vi "网分测量.vi"() -> (2 "Freq&S":T1)   [LabVIEW 2015]
uses:
  network_Global/Global.vi
  network/network.lvclass
  E5071C/Agilent ENA Series/Agilent ENA Series.lvlib
panel:
  in  "VISA resource name":refnum<visa-resource-name>
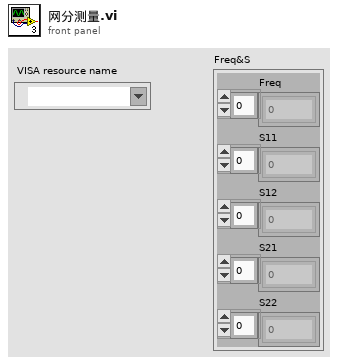
[diagram p1: front panel]
types:
  T1 = cluster{"Freq":dbl[], "S11":dbl[], "S12":dbl[], "S21":dbl[], "S22":dbl[]}
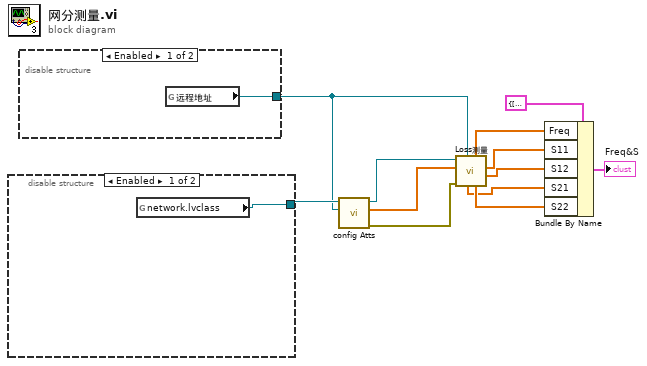
[diagram p0: block diagram]
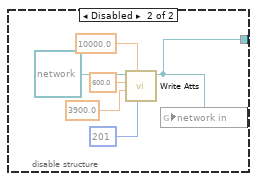
[diagram p2: hidden frame]
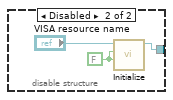
[diagram p3: hidden frame]
diagram:
  n1 = disable-structure shown="Enabled" {
    disable-tunnel: [w13 w14] -> w10
    frame Enabled {
      n2 = global read "Global.vi" "network.lvclass"() -> (w13:refnum<class "network.lvclass">)
    }
    frame Disabled {
      n3 = call-dynamic "Write Atts.vi"("Points"=201, "IF_Band"=10000.0, "Stop"=3900.0 ("Start"), "Start"=600.0, "network in"=refnum<class "network.lvclass"> refnum ("network.lvclass")) -> ("network out"=w14:refnum<class "network.lvclass">)  [unwired: 5 in, 1 out]
      n4 = global write "Global.vi" "network in"(w14) -> ()
    }
  }
  n5 = disable-structure shown="Enabled" {
    disable-tunnel: [w20 w21] -> w6
    frame Enabled {
      n6 = global read "Global.vi" "远程地址"() -> (w20:refnum<visa-resource-name>)
    }
    frame Disabled {
      w23 = FALSE ("Reset? (T: Yes)")
      n7 = call "Initialize.vi"("Reset? (T: Yes)"=w23, "ID Query? (T: Yes)"=w23, "VISA resource name"="VISA resource name") -> ("VISA resource name out"=w21:refnum<visa-resource-name>)  [unwired: 7 in, 1 out]
    }
  }
  n8 = call-dynamic "config Atts.vi"("VISA resource name"=w6, "network in"=w10) -> ("error out"=w9:errorcluster, "Freq"=w8:dbl[], "network out"=w7:refnum<class "network.lvclass">)  [unwired: 7 in]
  n9 = call-dynamic "Loss测量.vi"("VISA resource name"=w6, "error in (no error)"=w9, "Freq"=w8, "network in"=w7) -> ("S12"=w3:dbl[], "S11"=w4:dbl[], "S22"=w2:dbl[], "freq"=w5:dbl[], "S21"=w1:dbl[])  [unwired: 1 in, 2 out]
  n10 = Bundle By Name(cluster=T1 {"Freq"=[], "S11"=[], "S12"=[], "S21"=[], "S22"=[]} ("Cluster"), "Freq"=w5, "S11"=w4, "S12"=w3, "S21"=w1, "S22"=w2) -> (→"Freq&S":T1)
